vi "TDC_DAQV26_Paralled_muon.vi"(8 "error in (no error)":errorcluster, 9 "stop":bool, 10 "save data":bool=TRUE, 11 "SMA mode":bool=TRUE) -> (3 "rate":dbl=1.039685324035924)   [LabVIEW 2017]
uses:
  <vilib>/Utility/file.llb/Write Delimited Spreadsheet (DBL).vi
  <vilib>/Utility/file.llb/Write Delimited Spreadsheet (I64).vi
panel:
  out "substring 3":string
  out "fine 2":u64=218864601 format="%x"
  out "substring 2":string
  out "concatenated string 2":string="#"
  out "hex integer string 2":string="23"
  out "x-y":i32=35
  out "substring":string
  in  "gps":bool
  out "hex integer string":string="07E8"
  out "Year":string="2024"
  out "error out 3":errorcluster
  in  "factor":i32=128
  in  "displayCR":bool=TRUE
  in  "Counter Setting":dbl=100000.0 format="%#_13g"
  in  "replace dat":bool
  in  "append csv":bool=TRUE
  in  "concatenated string":string="Z\u000f"
  out "number":u32=35
  out "element":string
  out "fine":u64=197 format="%x"
  in  "UDP Config":bool=TRUE
  in  "data  path":path=path "G:/tdc/2017"
  out "cal 2":u64[](graph)
  in  "Thresholds (mV)":u16[](array[numeric])=[580, 580, 580, 580, 600, 600, 600, 600, 580, 580, 600, 600, 600, 600, 600, 600, 580, 580, 600, 600, 600, 600, 600, 600, 580, 580, 600, 600, 600, 600, 600, 600]
  out "error out 2":errorcluster={"status"=TRUE, "code"=1, "source"="Dequeue Element in TDC_DAQV26_Paralled_muon.vi"}
  in  "display":bool=TRUE
  in  "Thresholds":u16=580
  in  "one key for threshold":bool=TRUE
  in  "RST":bool
  in  "通道数量":i32=128
  out "Cal Table":u32[](array[numeric])=[100002, 100002, 100002, 100002, 100002, 100002, 100002, 100002, 100002, 100002, 100002, 100002, 100002, 100002, 100002, 100002, 100002, 100002, 100002, 100002, 100002, 100002, 100002, 100002, 100002, 100002, 100002, 100002, 100002, 100002, 100002, 100002, 100002, 0, 0, 0, 100002, 0, 0, 0, 0, 0, 0, 0, 0, 0, 0, 0, 0, 0, 0, 0, 0, 0, 0, 0, 0, 0, 0, 0, 0, 0, 0, 0, 0, 0, 0, 0, 0, 0, 0, 0, 0, 0, 0, 0, 0, 0, 0, 0, 0, 0, 0, 0, 0, 0, 0, 0, 0, 0, 0, 0, 0, 0, 0, 0, 0, 0, 0, 0, 0, 0, 0, 0, 0, 0, 0, 0, 0, 0, 0, 0, 0, 0, 0, 0, 0, 0, 0, 0, 0, 0, 0, 0, 0, 0, 0, 0]
  in  "channel for cal":i32
  out "channel number":u64=10
  in  "bytes to read":i32=320
  out "Calibration Counter":i32=100000
  out "Event index":i32=97959
  out "cal":u32[](graph)=[0, 0, 0, 0, 0, 0, 0, 0, 0, 0, 0, 0, 0, 0, 0, 0, 0, 0, 0, 0, 0, 0, 0, 0, 0, 0, 0, 0, 0, 0, 0, 0, 0, 0, 0, 0, 0, 0, 0, 0, 0, 0, 0, 0, 0, 0, 0, 0, 0, 0, 0, 0, 0, 0, 0, 0, 0, 0, 0, 0, 0, 0, 0, 0, 0, 0, 0, 0, 0, 0, 0, 0, 0, 0, 0, 0, 0, 0, 0, 0, 0, 0, 0, 0, 0, 0, 0, 0, 0, 0, 0, 0, 0, 0, 0, 0, 0, 0, 0, 0, 0, 0, 0, 0, 0, 0, 0, 0, 0, 0, 0, 0, 0, 0, 0, 0, 0, 0, 0, 0, 0, 0, 0, 0, 0, 0, 0, 0, 0, 0, 0, 0, 0, 0, 0, 0, 0, 0, 0, 0, 0, 0, 0, 0, 0, 0, 0, 0, 0, 0, 0, 0, 0, 0, 0, 0, 0, 0, 0, 10, 71, 320, 55, 788, 157, 172, 696, 64, 82, 262, 173, 135, 530, 87, 255, 177, 53, 608, 293, 326, 71, 47, 118, 254, 336, 311, 104, 51, 60, 101, 372, 166, 178, 168, 245, 175, 255, 440, 146, 44, 45, 205, 363, 299, 66, 85, 64, 46, 161, 73, 87, 47, 79, 666, 246, 61, 75, 55, 178, 83, 250, 291, 46, 49, 206, 160, 459, 68, 164, 175, 127, 374, 157, 65, 63, 140, 125, 65, 81, 86, 171, 166, 294, 130, 57, 56, 35, 61, 101, 38, 351, 101, 459, 108, 74, 68, 117, 70, 135, 136, 194, 46, 513, 47, 37, 299, 54, 123, 69, 303, 46, 39, 36, 153, 122, 350, 130, 86, 162, 135, 148, 117, 311, 184, 79, 167, 252, 57, 123, 76, 268, 69, 54, 100, 252, 57, 39, 66, 495, 175, 138, 53, 162, 69, 123, 49, 63, 111, 337, 184, 50, 101, 59, 156, 75, 54, 232, 351, 53, 241, 137, 45, 169, 83, 112, 45, 278, 398, 106, 103, 61, 225, 114, 53, 349, 136, 144, 139, 230, 47, 41, 39, 128, 264, 88, 328, 63, 460, 373, 100, 51, 59, 290, 101, 576, 134, 101, 92, 70, 72, 60, 138, 192, 163, 185, 250, 92, 55, 83, 85, 80, 179, 133, 107, 81, 386, 79, 65, 147, 96, 111, 306, 281, 141, 140, 234, 96, 322, 73, 54, 60, 107, 284, 77, 115, 71, 69, 168, 320, 56, 166, 190, 154, 153, 95, 120, 232, 147, 59, 47, 78, 316, 84, 44, 84, 412, 156, 67, 173, 188, 56, 93, 78, 172, 586, 79, 69, 63, 47, 30, 64, 176, 76, 99, 504, 173, 60, 57, 150, 175, 76, 54, 70, 88, 41, 519, 208, 91, 467, 49, 53, 40, 46, 371, 122, 142, 66, 216, 120, 48, 56, 64, 174, 362, 68, 302, 82, 78, 72, 347, 92, 85, 188, 270, 100, 62, 123, 182, 178, 324, 127, 165, 107, 189, 184, 56, 252, 122, 111, 123, 54, 240, 39, 50, 87, 353, 187, 265, 56, 49, 52, 48, 128, 342, 202, 83, 124, 111, 57, 70, 215, 119, 215, 90, 61, 159, 220, 46, 92, 225, 254, 104, 89, 54, 63, 93, 57, 49, 59, 794, 66, 46, 60, 66, 62, 331, 151, 145, 387, 94, 133, 45, 205, 163, 301, 70, 138, 341, 53, 361, 46, 47, 68, 64, 302, 126, 52, 31, 77, 86, 107, 236, 304, 50, 48, 82, 126, 116, 287, 66, 89, 80, 166, 51, 64, 238, 179, 185, 64, 408, 113, 149, 102, 141, 66, 247, 73, 343, 243, 108, 99, 64, 283, 309, 137, 95, 347, 128, 229, 519, 63, 378, 71, 121, 342, 558, 83, 91, 138, 114, 155, 93, 202, 215, 179, 311, 80, 108, 142, 151, 209, 117, 114, 100, 128, 194, 185, 423, 207, 173, 217, 105, 119, 114, 321, 92, 139, 114, 73, 159, 67, 91, 311, 77, 144, 150, 323, 241, 221, 146, 174, 293, 75, 57, 79, 130, 288, 72, 123, 113, 361, 224, 84, 135, 88, 118, 155, 184, 119, 62, 88, 114, 62, 186, 97, 52, 234, 165, 49, 71, 72, 195, 364, 217, 84, 63, 64, 73, 162, 227, 133, 507, 60, 197, 272, 61, 49, 160, 197, 89, 89, 128, 107, 117, 177, 163, 91, 114, 57, 64, 219, 83, 119, 170, 56, 77, 56, 67, 218, 120, 281, 171, 136, 159, 61, 43, 105, 74, 126, 202, 159, 98, 320, 66, 105, 324, 210, 151, 79, 81, 115, 144, 148, 470, 209, 115, 114, 121, 116, 138, 158, 349, 112, 170, 362, 161, 214, 209, 170, 130, 131, 389, 42, 175, 208, 68, 128, 313, 195, 123, 303, 45, 253, 76, 73, 95, 254, 197, 55, 99, 114, 169, 141, 377, 223, 106, 53, 121, 137, 49, 56, 57, 46, 138, 258, 58, 83, 123, 67, 62, 147, 76, 33, 67, 174, 25, 16, 19, 20, 39, 20, 82, 17, 24, 72, 21, 8, 21, 21, 10, 2, 6, 6, 3, 0, 2, 0, 0, 0, 0, 0, 0, 0, 0, 0, 0, 0, 0, 0, 0, 0, 0, 0, 0, 0, 0, 0, 0, 0, 0, 0, 0, 0, 0, 0, 0, 0, 0, 0, 0, 0, 0, 0, 0, 0, 0, 0, 0, 0, 0, 0, 0, 0, 0, 0, 0, 0, 0, 0, 0, 0, 0, 0, 0, 0, 0, 0, 0, 0, 0, 0, 0, 0, 0, 0, 0, 0, 0, 0, 0, 0, 0, 0, 0, 0, 0, 0, 0, 0, 0, 0, 0, 0, 0, 0, 0, 0, 0, 0, 0, 0, 0, 0, 0, 0, 0, 0, 0, 0, 0, 0, 0, 0, 0, 0, 0, 0, 0, 0, 0, 0, 0, 0, 0, 0, 0, 0, 0, 0, 0, 0, 0, 0, 0, 0, 0, 0, 0, 0, 0, 0, 0, 0, 0, 0, 0, 0, 0, 0, 0, 0, 0, 0, 0, 0, 0, 0, 0, 0, 0, 0, 0, 0, 0, 0, 0, 0, 0, 0, 0, 0, 0, 0, 0, 0, 0, 0, 0, 0, 0, 0, 0, 0, 0, 0, 0, 0, 0, 0, 0, 0, 0, 0, 0, 0, 0, 0, 0, 0, 0, 0, 0, 0, 0, 0, 0, 0, 0, 0, 0, 0, 0, 0, 0, 0, 0, 0, 0, 0, 0, 0, 0, 0, 0, 0, 0, 0, 0, 0, 0, 0, 0, 0, 0, 0, 0, 0, 0, 0, 0, 0, 0, 0, 0, 0, 0, 0, 0, 0, 0, 0, 0, 0, 0, 0, 0, 0, 0, 0, 0, 0, 0, 0, 0, 0, 0, 0, 0, 0, 0, 0, 0, 0, 0, 0, 0, 0, 0, 0, 0, 0, 0, 0, 0, 0, 0, 0, 0, 0, 0, 0, 0, 0, 0, 0, 0, 0, 0, 0, 0, 0, 0, 0, 0, 0, 0, 0, 0, 0, 0, 0, 0, 0, 0, 0, 0, 0, 0, 0, 0, 0, 0, 0, 0, 0, 0, 0, 0, 0, 0, 0, 0, 0, 0, 0, 0, 0, 0, 0, 0, 0, 0, 0, 0, 0, 0, 0, 0, 0, 0, 0, 0, 0, 0, 0, 0, 0, 0, 0, 0, 0, 0, 0, 0, 0, 0, 0, 0, 0, 0, 0, 0, 0, 0, 0, 0, 0, 0, 0, 0, 0, 0, 0, 0, 0, 0, 0, 0, 0, 0, 0, 0, 0, 0, 0, 0, 0, 0, 0, 0, 0, 0, 0, 0, 0, 0, 0, 0, 0, 0, 0, 0, 0, 0, 0, 0, 0, 0, 0, 0, 0, 0, 0, 0, 0, 0, 0, 0, 0, 0, 0, 0, 0, 0, 0, 0, 0, 0, 0, 0, 0, 0, 0, 0, 0, 0, 0, 0, 0, 0, 0, 0, 0, 0, 0, 0, 0, 0, 0, 0, 0, 0, 0, 0, 0, 0, 0, 0, 0, 0, 0, 0, 0, 0, 0, 0, 0, 0, 0, 0, 0, 0, 0, 0, 0, 0, 0, 0, 0, 0, 0, 0, 0, 0, 0, 0, 0, 0, 0, 0, 0, 0, 0, 0, 0, 0, 0, 0, 0, 0, 0, 0, 0, 0, 0, 0, 0, 0, 0, 0, 0, 0, 0, 0, 0, 0, 0, 0, 0, 0, 0, 0, 0, 0, 0, 0, 0, 0, 0, 0, 0, 0, 0, 0, 0, 0, 0, 0, 0, 0, 0, 0, 0, 0, 0, 0, 0, 0, 0, 0, 0, 0, 0, 0, 0, 0, 0, 0, 0, 0, 0, 0, 0, 0, 0, 0, 0, 0, 0, 0, 0, 0, 0, 0, 0, 0, 0, 0, 0, 0, 0, 0, 0, 0, 0, 0, 0, 0, 0, 0, 0, 0, 0, 0, 0, 0, 0, 0, 0, 0, 0, 0, 0, 0, 0, 0, 0, 0, 0, 0, 0, 0, 0, 0, 0, 0, 0, 0, 0, 0, 0, 0, 0, 0, 0, 0, 0, 0, 0, 0, 0, 0, 0, 0, 0, 0, 0, 0, 0, 0, 0, 0, 0, 0, 0, 0, 0, 0, 0, 0, 0, 0, 0, 0, 0, 0, 0, 0, 0, 0, 0, 0, 0, 0, 0, 0, 0, 0, 0, 0, 0, 0, 0, 0, 0, 0, 0, 0, 0, 0, 0, 0, 0, 0, 0, 0, 0, 0, 0, 0, 0, 0, 0, 0, 0, 0, 0, 0, 0, 0, 0, 0, 0, 0, 0, 0, 0, 0, 0, 0, 0, 0, 0, 0, 0, 0, 0, 0, 0, 0, 0, 0, 0, 0, 0, 0, 0, 0, 0, 0, 0, 0, 0, 0, 0, 0, 0, 0, 0, 0, 0, 0, 0, 0, 0, 0, 0, 0, 0, 0, 0, 0, 0, 0, 0, 0, 0, 0, 0, 0, 0, 0, 0, 0, 0, 0, 0, 0, 0, 0, 0, 0, 0, 0, 0, 0, 0, 0, 0, 0, 0, 0, 0, 0, 0, 0, 0, 0, 0, 0, 0, 0, 0, 0, 0, 0, 0, 0, 0, 0, 0, 0, 0, 0, 0, 0, 0, 0, 0, 0, 0, 0, 0, 0, 0, 0, 0, 0, 0, 0, 0, 0, 0, 0, 0, 0, 0, 0, 0, 0, 0, 0, 0, 0, 0, 0, 0, 0, 0, 0, 0, 0, 0, 0, 0, 0, 0, 0, 0, 0, 0, 0, 0, 0, 0, 0, 0, 0, 0, 0, 0, 0, 0, 0, 0, 0, 0, 0, 0, 0, 0, 0, 0, 0, 0, 0, 0, 0, 0, 0, 0, 0, 0, 0, 0, 0, 0, 0, 0, 0, 0, 0, 0, 0, 0, 0, 0, 0, 0, 0, 0, 0, 0, 0, 0, 0, 0, 0, 0, 0, 0, 0, 0, 0, 0, 0, 0, 0, 0, 0, 0, 0, 0, 0, 0, 0, 0, 0, 0, 0, 0, 0, 0, 0, 0, 0, 0, 0, 0, 0, 0, 0, 0, 0, 0, 0, 0, 0, 0, 0, 0, 0, 0, 0, 0, 0, 0, 0, 0, 0, 0, 0, 0, 0, 0, 0, 0, 0, 0, 0, 0, 0, 0, 0, 0, 0, 0, 0, 0, 0, 0, 0, 0, 0, 0, 0, 0, 0, 0, 0, 0, 0, 0, 0, 0, 0, 0, 0, 0, 0, 0, 0, 0, 0, 0, 0, 0, 0, 0, 0, 0, 0, 0, 0, 0, 0, 0, 0, 0, 0, 0, 0, 0, 0, 0, 0, 0, 0, 0, 0, 0, 0, 0, 0, 0, 0, 0, 0, 0, 0, 0, 0, 0, 0, 0, 0, 0, 0, 0, 0, 0, 0, 0, 0, 0, 0, 0, 0, 0, 0, 0, 0, 0, 0, 0, 0, 0, 0, 0, 0, 0, 0, 0, 0, 0, 0, 0, 0, 0, 0, 0, 0, 0, 0, 0, 0, 0, 0, 0, 0, 0, 0, 0, 0, 0, 0, 0, 0, 0, 0, 0, 0, 0, 0, 0, 0, 0, 0, 0, 0, 0, 0, 0, 0, 0, 0, 0, 0, 0, 0, 0, 0, 0, 0, 0, 0, 0, 0, 0, 0, 0, 0, 0, 0, 0, 0, 0, 0, 0, 0, 0, 0, 0, 0, 0, 0, 0, 0, 0, 0, 0, 0, 0, 0, 0, 0, 0, 0, 0, 0, 0, 0, 0, 0, 0, 0, 0, 0, 0, 0, 0, 0, 0, 0, 0, 0, 0, 0, 0, 0, 0, 0, 0, 0, 0, 0, 0, 0, 0, 0, 0, 0, 0, 0, 0, 0, 0, 0, 0, 0, 0, 0, 0, 0, 0, 0, 0, 0, 0, 0, 0, 0, 0, 0, 0, 0, 0, 0]
  out "error out":errorcluster
  out "appended path":path=path "G:/tdc/2017/test_20241217_115315.dat"
  in  "filename":string="test"
  in  "Events":i32=110000 min=1
  in  "timeout (ms)":i32=10000
  in  "address":string="192.168.10.35"
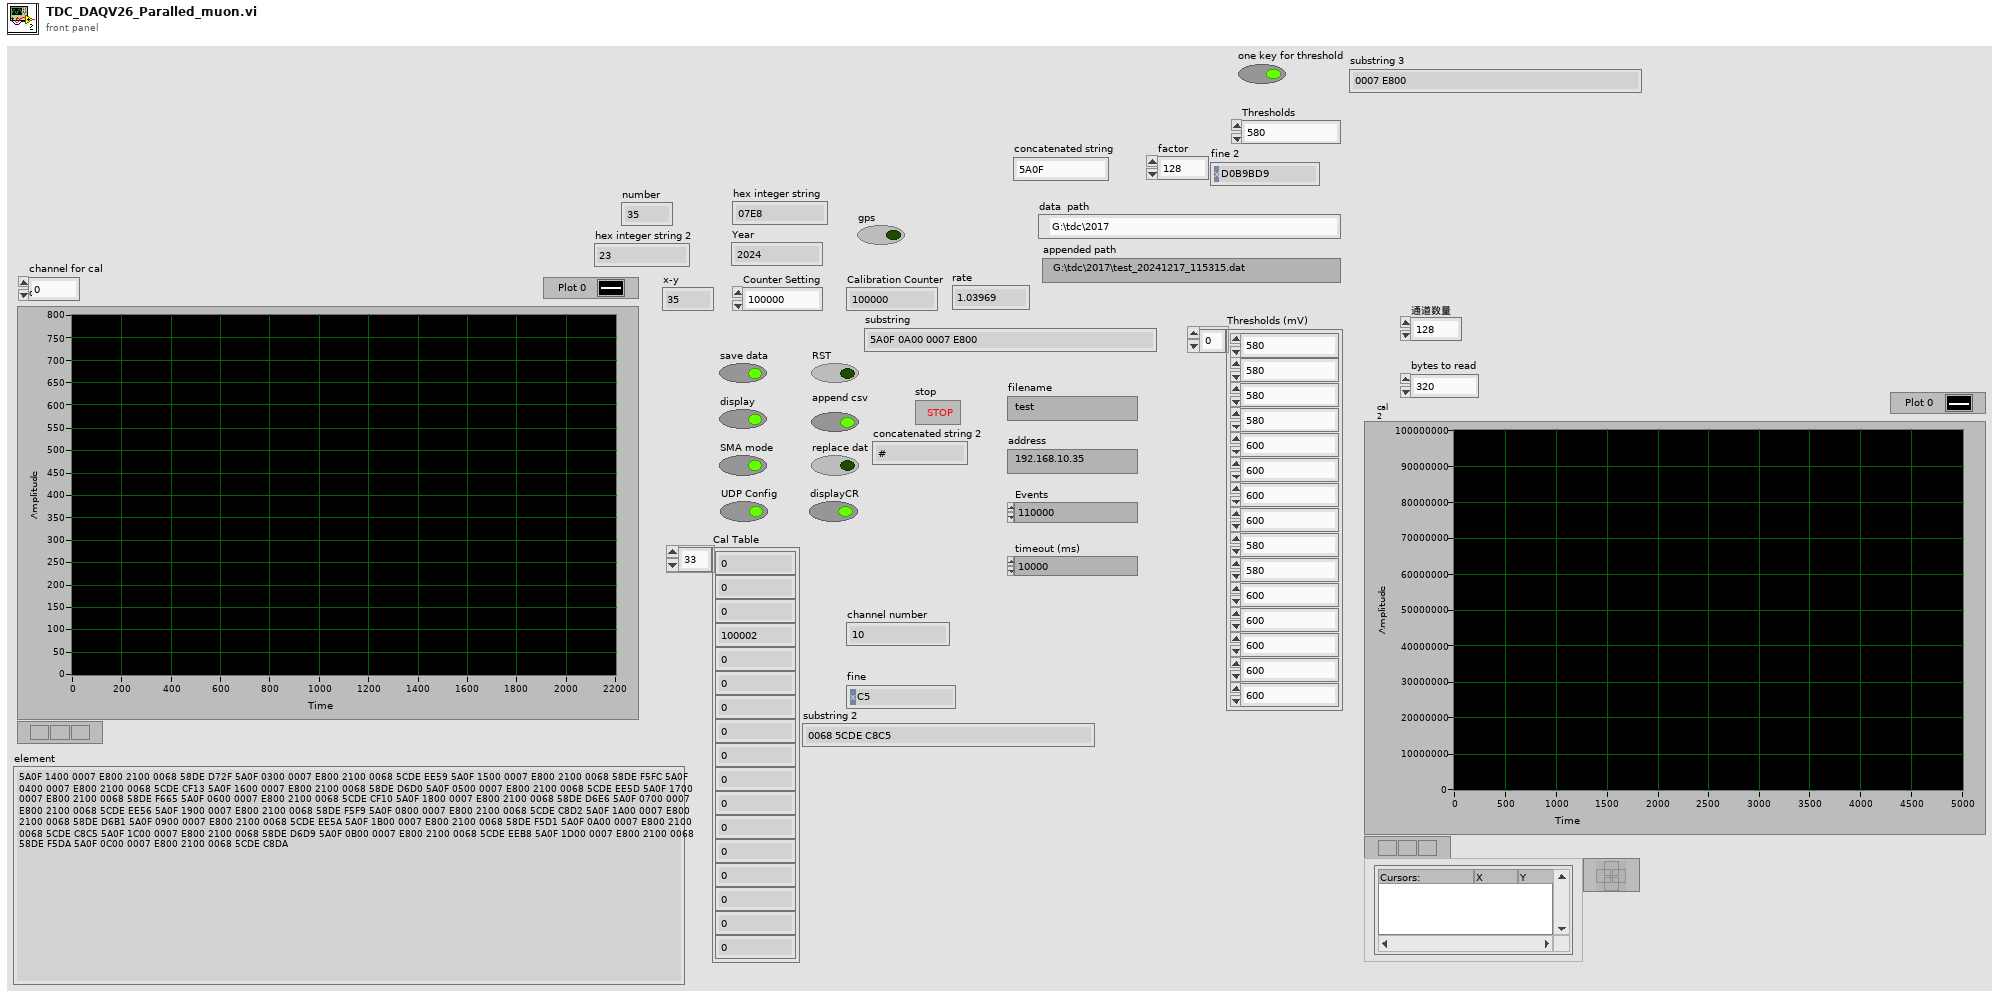
[diagram p1: front panel]
types:
  T1 = enum16{"open", "replace", "create", "open or create", "replace or create", "replace or create with confirmation"}
  T2 = enum16{"Standard", "Buffered", "CRLF", "Immediate"}
  T3 = enum16{"big-endian, network order", "native, host order", "little-endian"}
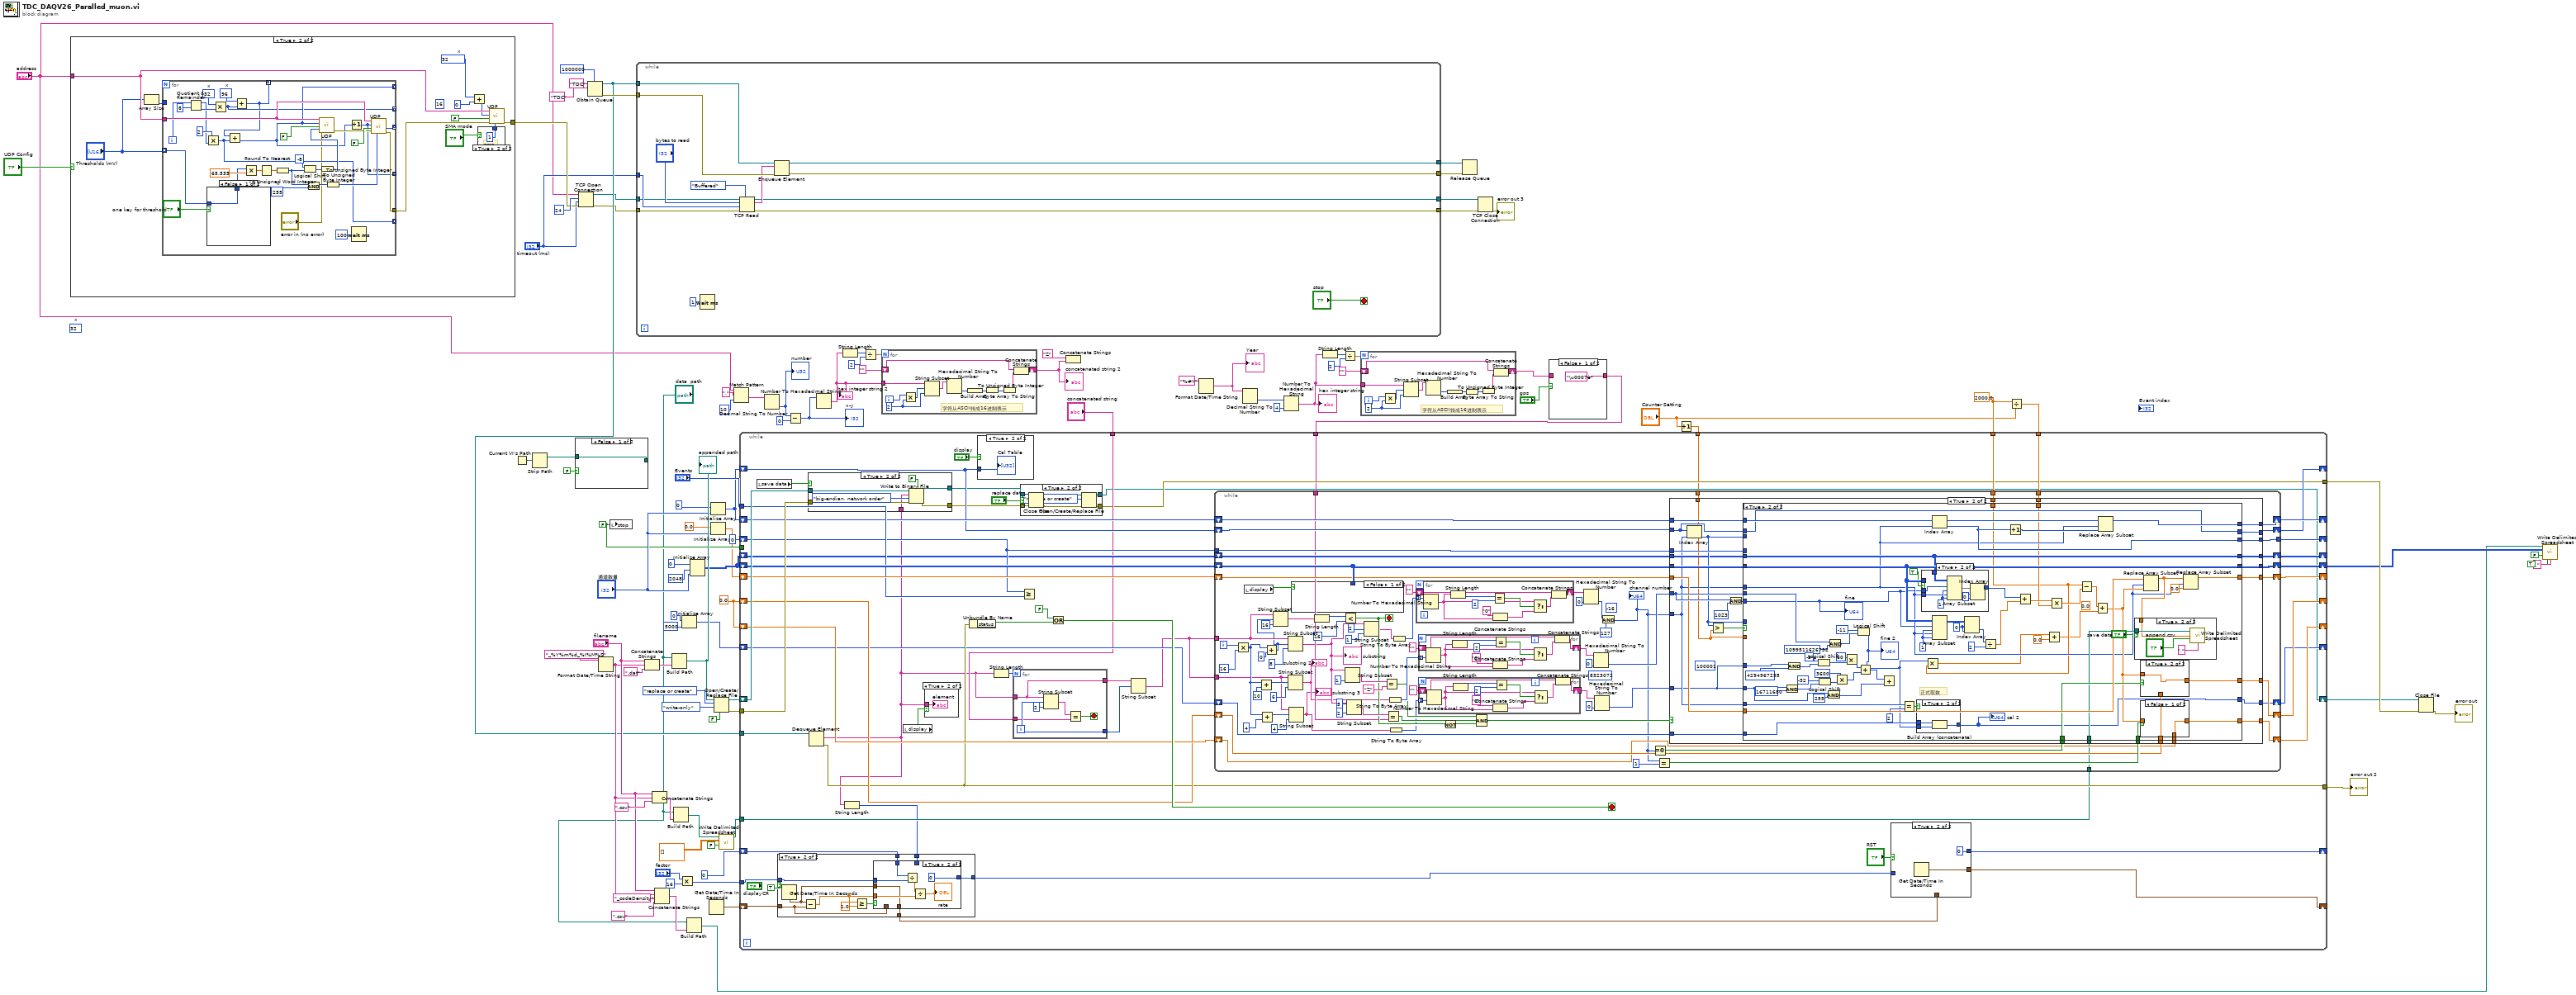
[diagram p0: block diagram]
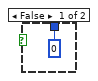
[diagram p4: hidden frame]
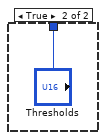
[diagram p5: hidden frame]
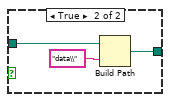
[diagram p6: hidden frame]
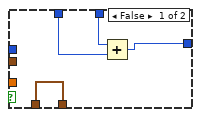
[diagram p11: hidden frame]
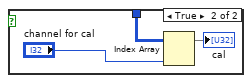
[diagram p14: hidden frame]
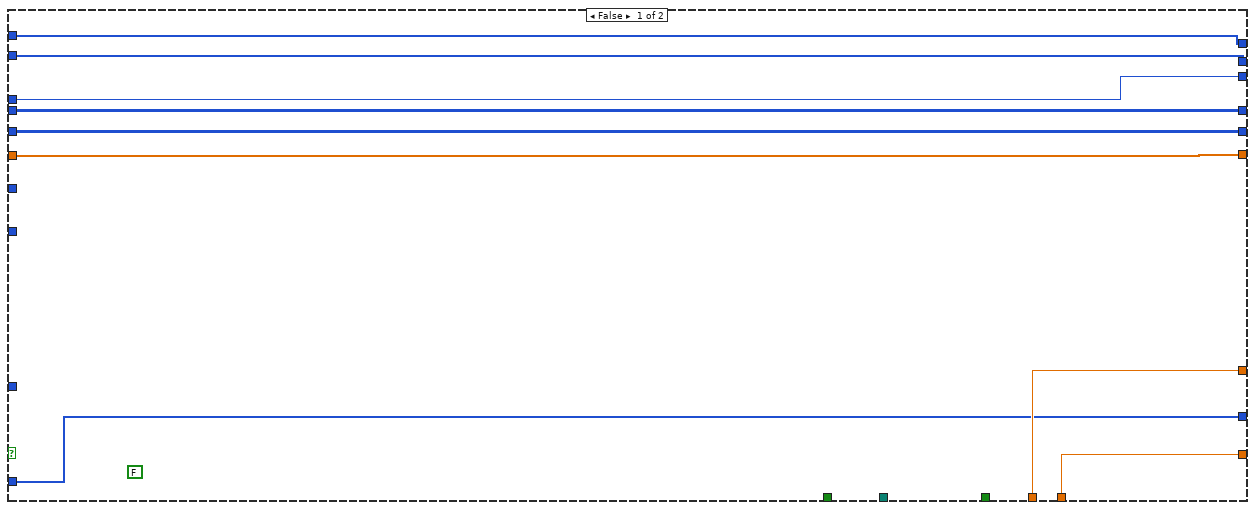
[diagram p15: hidden frame]
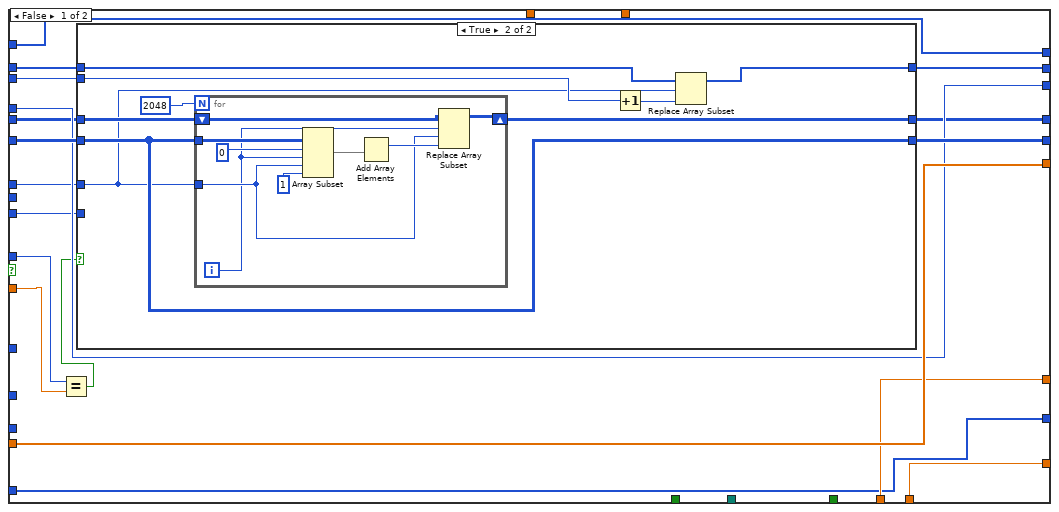
[diagram p16: hidden frame]
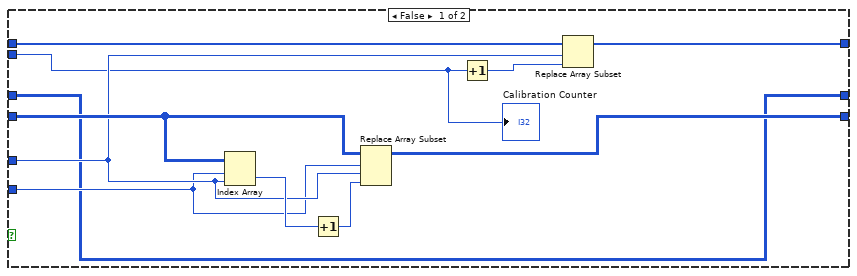
[diagram p17: hidden frame]
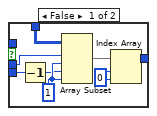
[diagram p20: hidden frame]
diagram:
  w26 = 2000.0 ("x")
  (unwired) u16 32  # x
  w68 = FALSE ("stop")
  w78 = 0.0
  n1 = case shown="True" "UDP Config" {
    tunnel: "address" -> [_ w111]
    tunnel: [_ w108] -> w69
    frame False {
    }
    frame True {
      (unwired) u32 16 ("Address")
      w102 = u16 32  # x
      n2 = Array Size(array="Thresholds (mV)") -> (size(s)=w105:i32)
      n3 = for {
        tunnel: w111 -> [w141]
        tunnel: "Thresholds (mV)" -> [w127] mode=indexing
        tunnel: [w135] -> _ mode=indexing
        tunnel: [w130] -> w109
        tunnel: w105 -> [_]
        tunnel: [w121] -> _ mode=indexing
        tunnel: [w120] -> _ mode=indexing
        tunnel: [w119] -> _ mode=indexing
        tunnel: [w118] -> _ mode=indexing
        tunnel: [w117] -> _ mode=indexing
        i -> [w122]
        w123 = u16 96  # x
        w124 = u16 32  # x
        w137 = u16 255  # x
        n4 = Quotient & Remainder(x=w122, y=8) -> (x-y*floor(x/y)=w116:i32, floor(x/y)=w125:i32)
        n5 = Multiply(x=2, y=w116) -> (x*y=w117:i32)
        n6 = case shown="False" "one key for threshold" {
          tunnel: [w147 "Thresholds"] -> w128
          tunnel: w127 -> [w147 _]
          frame False {
          }
          frame True {
          }
        }
        n7 = Multiply(x=w124, y=w125) -> (x*y=w119:i32)
        n8 = Add(x=w123, y=w119) -> (x+y=w118:i32)
        n9 = Add(x=w118, y=w117) -> (x+y=w121:i32)
        n10 = Multiply(x=w128, y=65.535) -> (x*y=w144:dbl)
        n11 = Round To Nearest(number=w144) -> (nearest integer value=w142:dbl)
        n12 = To Unsigned Word Integer(number=w142) -> (unsigned 16bit integer=w132:u16)
        n13 = Logical Shift(y=i16 -8, x=w132) -> (x << y=w139:u16)
        n14 = And(x=w132, y=w137) -> (x .and. y?=w136:u16)
        n15 = To Unsigned Byte Integer(number=w139) -> (unsigned 8bit integer=w138:u8)
        n16 = call "UDP.vi"("In"=w138, "error in (no error)"="error in (no error)", "Read (TRUE)"=FALSE, "Address"=w121, "IP address"=w141) -> ("error out"=w131:errorcluster)  [unwired: 4 in, 1 out]
        n17 = To Unsigned Byte Integer(number=w136) -> (unsigned 8bit integer=w134:u8)
        n18 = Increment(x=w121) -> (x+1=w120:i32)
        n19 = Wait (ms)(milliseconds to wait=u32 100) -> ()  [unwired: 1 out]
        n20 = call "UDP.vi"("In"=w134, "error in (no error)"=w131, "Read (TRUE)"=FALSE, "Address"=w120, "IP address"=w141) -> ("error out"=w130:errorcluster, "Out"=w135:u8)  [unwired: 4 in]
      }
      n21 = Add(x=w102, y=u32 0 ("Address")) -> (x+y=w101:u32)
      n22 = case shown="True" "SMA mode" {
        tunnel: [u8 0 ("In") u8 1 ("In")] -> w107
        frame False {
        }
        frame True {
          # "sma"
        }
      }
      n23 = call "UDP.vi"("In"=w107, "error in (no error)"=w109, "Read (TRUE)"=FALSE, "Address"=w101, "IP address"=w111) -> ("error out"=w108:errorcluster)  [unwired: 4 in, 1 out]
    }
  }
  n24 = Current VI's Path() -> (path=w94:path)
  n25 = Strip Path(path=w94) -> (stripped path=w93:path)  [unwired: 1 out]
  n26 = case shown="False" FALSE {
    tunnel: w93 -> [w149 w151]
    tunnel: [w149 w150] -> _
    frame False {
    }
    frame True {
      n27 = Build Path(base path=w151, name or relative path="data\\") -> (appended path=w150:path)
    }
  }
  n28 = TCP Open Connection(address="address", remote port or service name=u16 24 ("port"), timeout ms (60000)="timeout (ms)", error in (no error)=w69) -> (connection ID=w52:refnum<k5>, error out=w53:errorcluster)  [unwired: 1 in]
  n29 = Obtain Queue(max queue size (-1, unlimited)=1000000, name (unnamed)="TDC", element data type="TDC" ("name (unnamed)")) -> (queue out=w54:refnum<queue>, error out=w55:errorcluster)  [unwired: 2 in, 1 out]
  n30 = Format Date/Time String(time format string (%c)="_%Y%m%d_%I%M%S") -> (date/time string=w66:string)  [unwired: 2 in]
  n31 = local write "stop"(w68) -> ()
  n32 = while {
    tunnel: w54 -> [w166]
    tunnel: w55 -> [w165]
    tunnel: w53 -> [w163]
    tunnel: "timeout (ms)" -> [w162]
    tunnel: w52 -> [w161]
    tunnel: [w159] -> w51
    tunnel: [w158] -> w50
    tunnel: [w156] -> w49
    tunnel: [w155] -> w48
    stop <- "stop" stop-if-true
    n33 = Wait (ms)(milliseconds to wait=u32 1) -> ()  [unwired: 1 out]
    n34 = TCP Read(connection ID=w161, bytes to read="bytes to read", error in (no error)=w163, 7:T2."Buffered" ("mode (standard)"), 9:w162) -> (connection ID out=w159:refnum<k5>, data out=w160:string, error out=w158:errorcluster)
    n35 = Enqueue Element(queue=w166, element=w160, error in (no error)=w165) -> (queue out=w156:refnum<queue>, error out=w155:errorcluster)  [unwired: 1 in, 1 out]
  }
  n36 = Concatenate Strings("filename", w66, ".dat") -> (w92:string)
  n37 = Concatenate Strings("filename", w66, ".csv") -> (w80:string)
  n38 = Concatenate Strings("filename", w66, "_codeDensity" ("string"), ".csv") -> (w63:string)
  n39 = Build Path(base path="data  path", name or relative path=w92) -> (appended path=w91:path)
  "appended path" <- w91
  n40 = Build Path(base path="data  path", name or relative path=w80) -> (appended path=w75:path)
  n41 = Multiply(x="factor", y=16) -> (x*y=w19:i32)
  n42 = Initialize Array(u32 0 ("element"), 5000 ("dimension size")) -> (w42:u32[])
  n43 = Build Path(base path="data  path", name or relative path=w63) -> (appended path=w60:path)
  n44 = Initialize Array(u32 0 ("element"), 2048 ("dimension size"), "通道数量") -> (w77:u32[][])
  n45 = Get Date/Time In Seconds() -> (seconds since 1Jan1904=w70:timestamp)
  n46 = Initialize Array(u32 0 ("element"), "通道数量") -> (w79:u32[])
  n47 = Initialize Array(0.0, "通道数量") -> (w44:dbl[])
  n48 = Open/Create/Replace File(file path (use dialog)=w91, operation (0:open)=T1."replace or create", access (0:read/write)=enum16{"read/write", "read-only", "write-only"}."write-only", disable buffering (F)=FALSE) -> (refnum out=w96:refnum<file>, error out=w95:errorcluster)  [unwired: 2 in, 1 out]
  n49 = call-poly <vilib>:"Write Delimited Spreadsheet.vi"("file path (dialog if empty)"=w75, "2D data"=dbl[][] [], "append to file? (new file:F)"=FALSE) -> ("new file path (Not A Path if cancelled)"=w74:path)  [unwired: 11 in, 1 out]
  n50 = Match Pattern(string="address", regular expression="." ("search string"), offset (0)=10) -> (after substring=w31:string)  [unwired: 3 out]
  n51 = Decimal String To Number(string=w31) -> (number=w3:i32)  [unwired: 2 in, 1 out]
  "number" <- w3
  n52 = Subtract(x=w3, y=0) -> (x-y=w2:i32)
  "x-y" <- w2
  n53 = Number To Hexadecimal String(2:w2) -> (0:w29:string)  [unwired: 1 in]
  "hex integer string 2" <- w29
  n54 = String Length(string=w29) -> (length=w36:i32)
  n55 = Divide(x=w36, y=2) -> (x/y=w37:dbl)
  n56 = for {
    N: w37 -> [_]
    shift-right: [w177] -> w1
    shift-left: "" ("format string") -> [w176]
    tunnel: w29 -> [w167]
    i -> [w175]
    w169 = 2 ("y")
    # "字符从ASCII转成16进制表示"
    n57 = Multiply(x=w175, y=w169) -> (x*y=w168:i32)
    n58 = String Subset(string=w167, offset (0)=w168, length (rest)=w169) -> (substring=w170:string)
    n59 = Hexadecimal String To Number(string=w170) -> (number=w174:u32)  [unwired: 2 in, 1 out]
    n60 = Build Array(w174) -> (w173:u32[])
    n61 = To Unsigned Byte Integer(number=w173) -> (unsigned 8bit integer=w172:u8[])
    n62 = Byte Array To String(unsigned byte array=w172) -> (string=w171:string)
    n63 = Concatenate Strings(w176, w171) -> (w177:string)
  }
  "concatenated string 2" <- w1
  n64 = Concatenate Strings("Z", w1) -> ()  [unwired: 1 out]
  n65 = Format Date/Time String(time format string (%c)="%#Y") -> (date/time string=w15:string)  [unwired: 2 in]
  "Year" <- w15
  n66 = Decimal String To Number(string=w15) -> (number=w14:i32)  [unwired: 2 in, 1 out]
  n67 = Number To Hexadecimal String(1:i16 4 ("width (-)"), 2:w14) -> (0:w8:string)
  "hex integer string" <- w8
  n68 = String Length(string=w8) -> (length=w10:i32)
  n69 = Divide(x=w10, y=2) -> (x/y=w11:dbl)
  n70 = for {
    N: w11 -> [_]
    shift-right: [w188] -> w7
    shift-left: "" ("format string") -> [w187]
    tunnel: w8 -> [w178]
    i -> [w186]
    w180 = 2 ("y")
    # "字符从ASCII转成16进制表示"
    n71 = Multiply(x=w186, y=w180) -> (x*y=w179:i32)
    n72 = String Subset(string=w178, offset (0)=w179, length (rest)=w180) -> (substring=w181:string)
    n73 = Hexadecimal String To Number(string=w181) -> (number=w185:u32)  [unwired: 2 in, 1 out]
    n74 = Build Array(w185) -> (w184:u32[])
    n75 = To Unsigned Byte Integer(number=w184) -> (unsigned 8bit integer=w183:u8[])
    n76 = Byte Array To String(unsigned byte array=w183) -> (string=w182:string)
    n77 = Concatenate Strings(w187, w182) -> (w188:string)
  }
  n78 = Release Queue(queue=w49, error in (no error)=w48) -> ()  [unwired: 1 in, 3 out]
  n79 = TCP Close Connection(connection ID=w51, error in (no error)=w50) -> (error out=→"error out 3":errorcluster)  [unwired: 1 in, 1 out]
  n80 = case shown="False" "gps" {
    tunnel: w7 -> [_ w190]
    tunnel: ["\u0007è" ("format string") w190] -> w6
    frame False {
    }
    frame True {
    }
  }
  n81 = Increment(x="Counter Setting") -> (x+1=w22:dbl)
  n82 = Divide(x=w26, y="Counter Setting") -> (x/y=w25:dbl)
  n83 = while {
    tunnel: w95 -> [w245]
    tunnel: [w219] -> w47
    tunnel: [w203] -> w88
    shift-right: [w242] -> w61
    shift-left: w77 -> [w243]
    shift-right: [w228] -> _
    shift-left: w44 -> [w241]
    tunnel: "Events" -> [w239]
    shift-right: [w238] -> _
    shift-left: w79 -> [w237]
    shift-right: [w236] -> _
    shift-left: u32 0 ("element") -> [w235]
    shift-right: [w234] -> _
    shift-left: w79 -> [w221]
    shift-right: [w233] -> _
    shift-left: w78 -> [w230]
    shift-right: [w232] -> _
    shift-left: w78 -> [w231]
    shift-right: [w223] -> _
    shift-left: w77 -> [w229]
    tunnel: w74 -> [w215]
    shift-right: [w227] -> _
    shift-left: 0 -> [w197]
    shift-right: [w225] -> _
    shift-left: w70 -> [w224]
    tunnel: w68 -> [_]
    tunnel: w54 -> [w220]
    shift-right: [w216] -> _
    shift-left: w42 -> [w217]
    tunnel: "concatenated string" -> [w211]
    tunnel: w26 -> [w209]
    tunnel: w25 -> [w208]
    shift-right: [w202] -> w24
    shift-left: w96 -> [w244]
    tunnel: w22 -> [w201]
    tunnel: w19 -> [w194]
    tunnel: w6 -> [w191]
    stop <- w240 stop-if-true
    n84 = local read "save data"() -> (w196:bool)
    n85 = Dequeue Element(queue=w220) -> (element=w207:string, error out=w219:errorcluster)  [unwired: 2 in, 2 out]
    n86 = case shown="True" w196 {
      tunnel: w245 -> [w247 w255]
      tunnel: w244 -> [w248 w254]
      tunnel: w207 -> [_ w251]
      tunnel: [w248 w250] -> w206
      tunnel: [w247 w249] -> w204
      frame False {
      }
      frame True {
        n87 = Write to Binary File(file (use dialog)=w254, data=w251, error in=w255, 5:FALSE ("prepend array or string size? (T)"), 9:T3."big-endian, network order" ("byte order (0:big-endian, network order)")) -> (refnum out=w250:refnum<file>, error out=w249:errorcluster)  [unwired: 1 in, 1 out]
      }
    }
    n88 = String Length(string=w207) -> (length=w198:i32)
    n89 = case shown="True" TRUE {
      tunnel: w224 -> [w272 w277]
      tunnel: [w272 w278] -> w200
      tunnel: w197 -> [w271 w276]
      tunnel: w198 -> [_ w275]
      tunnel: [w271 w274] -> w199
      tunnel: w194 -> [_ w273]
      frame False {
      }
      frame True {
        n90 = Get Date/Time In Seconds() -> (seconds since 1Jan1904=w279:timestamp)
        n91 = Subtract(x=w279, y=w277) -> (x-y=w281:dbl)
        n92 = Greater Or Equal?(x=w281, y=1.0) -> (x >= y?=w282:bool)
        n93 = case shown="True" w282 {
          tunnel: w281 -> [_ w293]
          tunnel: w279 -> [_ w291]
          tunnel: [w286 w291] -> w278
          tunnel: w277 -> [w286 _]
          tunnel: w276 -> [w285 w288]
          tunnel: w275 -> [w284 _]
          tunnel: [w283 0] -> w274
          tunnel: w273 -> [_ w287]
          frame False {
            n94 = Add(x=w284, y=w285) -> (x+y=w283:i32)
          }
          frame True {
            n95 = Divide(x=w288, y=w287) -> (x/y=w290:dbl)
            n96 = Divide(x=w290, y=w293) -> (x/y=→"rate":dbl)
          }
        }
      }
    }
    n97 = local read "display"() -> (w195:bool)
    n98 = case shown="True" w195 {
      tunnel: w207 -> [_ w246]
      frame False {
      }
      frame True {
        "element" <- w246
      }
    }
    n99 = Unbundle By Name(w219) -> ("status"=w218:bool)
    n100 = case shown="True" "display" {
      tunnel: w221 -> [_ w294]
      frame False {
      }
      frame True {
        "Cal Table" <- w294
      }
    }
    n101 = String Length(string=w207) -> (length=w214:i32)
    n102 = for {
      N: w214 -> [_]
      tunnel: w207 -> [w267]
      tunnel: [w267] -> w213
      tunnel: [w266] -> w212
      tunnel: w211 -> [w265]
      i -> [w266]
      stop <- w268 stop-if-true
      n103 = String Subset(string=w267, offset (0)=w266, length (rest)=2 ("length (rest)")) -> (substring=w269:string)
      n104 = Equal?(x=w269, y=w265) -> (x = y?=w268:bool)
    }
    n105 = case shown="True" "replace dat" {
      tunnel: w206 -> [w257 w263]
      tunnel: [w257 w262] -> w202
      tunnel: w204 -> [w256 w259]
      tunnel: [w256 w258] -> w203
      frame False {
      }
      frame True {
        n106 = Close File(refnum=w263, error in=w259) -> (path=w264:path, error out=w260:errorcluster)
        n107 = Open/Create/Replace File(file path (use dialog)=w264, error in=w260, operation (0:open)=T1."replace or create") -> (refnum out=w262:refnum<file>, error out=w258:errorcluster)  [unwired: 3 in, 1 out]
      }
    }
    n108 = Greater Or Equal?(x=w235, y=w239) -> ()  [unwired: 1 out]
    n109 = Or(x=FALSE, y=w218) -> (x .or. y?=w240:bool)
    n110 = String Subset(string=w213, offset (0)=w212) -> (substring=w192:string)  [unwired: 1 in]
    n111 = while {
      tunnel: w192 -> [w325]
      shift-right: [w373] -> w242
      shift-left: w243 -> [w371]
      shift-right: [w369] -> w228
      shift-left: w241 -> [w370]
      shift-right: [w366] -> w238
      shift-left: w237 -> [w365]
      tunnel: [w364] -> w236
      tunnel: w235 -> [w363]
      shift-right: [w361] -> w234
      shift-left: w221 -> [w362]
      shift-right: [w357] -> w233
      shift-left: w230 -> [w355]
      shift-right: [w353] -> w232
      shift-left: w231 -> [w354]
      tunnel: w215 -> [w352]
      shift-right: [w351] -> w223
      shift-left: w229 -> [w319]
      shift-right: [w348] -> w216
      shift-left: w217 -> [w349]
      tunnel: w192 -> [w312]
      tunnel: w209 -> [w327]
      tunnel: w208 -> [w326]
      tunnel: w201 -> [w318]
      tunnel: w191 -> [w306]
      i -> [w374]
      stop <- w321 stop-if-true
      (unwired) u64 8323072 ("port")
      (unwired) i16 -16 ("y")
      n112 = Multiply(x=w374, y=16 ("length (rest)")) -> (x*y=w313:i32)
      n113 = local read "display"() -> (w350:bool)
      n114 = Add(x=w313, y=10 ("length (rest)")) -> (x+y=w340:i32)
      n115 = Add(x=w313, y=4 ("length (rest)")) -> (x+y=w315:i32)
      n116 = Add(x=w313, y=0 ("length (rest)")) -> (x+y=w324:i32)
      n117 = String Subset(string=w325, offset (0)=w324, length (rest)=16 ("y")) -> (substring=w322:string)
      n118 = String Subset(string=w325, offset (0)=w324, length (rest)=8 ("length (rest)")) -> (substring=w304:string)
      "substring" <- w304
      n119 = String Subset(string=w312, offset (0)=w340, length (rest)=6 ("length (rest)")) -> (substring=w300:string)
      "substring 2" <- w300
      n120 = String Subset(string=w312, offset (0)=w315, length (rest)=4 ("length (rest)")) -> (substring=w299:string)
      "substring 3" <- w299
      n121 = case shown="False" w350 {
        tunnel: w371 -> [_ w400]
        frame False {
        }
        frame True {
          n122 = Index Array(array=w400, index (col)="channel for cal") -> (element=→"cal":u32[])  [unwired: 1 in]
        }
      }
      n123 = String Length(string=w322) -> (length=w368:i32)
      n124 = Less?(x=w368, y=16) -> (x < y?=w321:bool)
      n125 = String Subset(string=w304, length (rest)=1 ("length (rest)")) -> (substring=w345:string)  [unwired: 1 in]
      n126 = String Subset(string=w304, offset (0)=5, length (rest)=2 ("length (rest)")) -> (substring=w328:string)
      n127 = String Subset(string=w304, offset (0)=2, length (rest)=1 ("length (rest)")) -> (substring=w302:string)
      n128 = Equal?(x=w345, y="Z" ("format string")) -> (x = y?=w330:bool)
      n129 = Equal?(x=w328, y=w306) -> (x = y?=w329:bool)
      n130 = String To Byte Array(string=w300) -> (unsigned byte array=w337:u8[])
      n131 = String To Byte Array(string=w299) -> (unsigned byte array=w308:u8[])
      n132 = String To Byte Array(string=w302) -> (unsigned byte array=w376:u8[])
      n133 = for {
        shift-right: [w588] -> w334
        shift-left: "" ("format string") -> [w585]
        tunnel: w376 -> [w589] mode=indexing
        n134 = Number To Hexadecimal String(2:w589) -> (0:w581:string)  [unwired: 1 in]
        n135 = String Length(string=w581) -> (length=w587:i32)
        n136 = Equal?(x=w587, y=2) -> (x = y?=w584:bool)
        n137 = Concatenate Strings("0" ("format string"), w581) -> (w583:string)
        n138 = Select(t=w581, s=w584, f=w583) -> (s? t:f=w580:string)
        n139 = Concatenate Strings(w585, w580) -> (w588:string)
      }
      n140 = for {
        shift-right: [w396] -> w335
        shift-left: "" ("format string") -> [w388]
        tunnel: w337 -> [w397] mode=indexing
        n141 = Number To Hexadecimal String(2:w397) -> (0:w390:string)  [unwired: 1 in]
        n142 = String Length(string=w390) -> (length=w395:i32)
        n143 = Concatenate Strings("0" ("format string"), w390) -> (w392:string)
        n144 = Equal?(x=w395, y=2) -> (x = y?=w393:bool)
        n145 = Select(t=w390, s=w393, f=w392) -> (s? t:f=w389:string)
        n146 = Concatenate Strings(w388, w389) -> (w396:string)
      }
      n147 = for {
        shift-right: [w386] -> w311
        shift-left: "" ("format string") -> [w378]
        tunnel: w308 -> [w387] mode=indexing
        n148 = Number To Hexadecimal String(2:w387) -> (0:w380:string)  [unwired: 1 in]
        n149 = String Length(string=w380) -> (length=w385:i32)
        n150 = Concatenate Strings("0" ("format string"), w380) -> (w382:string)
        n151 = Equal?(x=w385, y=2) -> (x = y?=w383:bool)
        n152 = Select(t=w380, s=w383, f=w382) -> (s? t:f=w379:string)
        n153 = Concatenate Strings(w378, w379) -> (w386:string)
      }
      n154 = Not(x=w321) -> (.not. x?=w320:bool)
      n155 = Compound Arithmetic op=AND(w330, w329, w320) -> (w343:bool)
      n156 = Hexadecimal String To Number(string=w334, default (0uL)=u64 0 ("default (0 U32)")) -> (number=w372:u64)  [unwired: 1 in, 1 out]
      n157 = Hexadecimal String To Number(string=w335, default (0uL)=u64 0 ("default (0 U32)")) -> (number=w333:u64)  [unwired: 1 in, 1 out]
      n158 = Hexadecimal String To Number(string=w311, default (0uL)=u64 0 ("default (0 U32)")) -> (number=w307:u64)  [unwired: 1 in, 1 out]
      n159 = And(x=w372, y=u64 127 ("port")) -> (x .and. y?=w301:u64)
      "channel number" <- w301
      n160 = Equal To 0?(x=w301) -> (x = 0?=w358:bool)
      n161 = Equal?(x=w301, y=u64 1) -> (x = y?=w356:bool)
      n162 = case shown="True" w343 {
        tunnel: w333 -> [_ w440]
        tunnel: w363 -> [w406 w430]
        tunnel: w371 -> [w409 w439]
        tunnel: [w409 w438] -> w373
        tunnel: [w408 w435] -> w369
        tunnel: w370 -> [w408 w434]
        tunnel: w301 -> [_ w414]
        tunnel: w365 -> [w407 w433]
        tunnel: [w407 w432] -> w366
        tunnel: [w406 w431] -> w364
        tunnel: w362 -> [w405 w429]
        tunnel: [w405 w428] -> w361
        tunnel: w358 -> [_ w427]
        tunnel: w355 -> [w404 w426]
        tunnel: [w404 w425] -> w357
        tunnel: w356 -> [_ w424]
        tunnel: w354 -> [w403 w423]
        tunnel: [w403 w422] -> w353
        tunnel: w319 -> [w402 w420]
        tunnel: [w402 w419] -> w351
        tunnel: w352 -> [_ w418]
        tunnel: w349 -> [w401 w416]
        tunnel: [w401 w415] -> w348
        tunnel: w327 -> [_ w413]
        tunnel: w326 -> [_ w412]
        tunnel: w318 -> [_ w411]
        tunnel: w307 -> [_ w410]
        frame False {
          (unwired) FALSE
        }
        frame True {
          (unwired) 100001 ("y")
          n163 = Index Array(array=w429, index=w414) -> (element=w421:u32)
          n164 = Greater?(x=w421, y=w411) -> (0:w417:bool)
          n165 = And(x=w440, y=u64 1023 ("port")) -> (x .and. y?=w436:u64)
          n166 = case shown="True" w417 {
            tunnel: w440 -> [_ w552]
            tunnel: w439 -> [w458 w538]
            tunnel: [w457 w538] -> w438
            tunnel: w436 -> [w449 w489]
            tunnel: [w456 w522] -> w435
            tunnel: w434 -> [w456 w545]
            tunnel: w430 -> [w454 _]
            tunnel: w414 -> [w452 w520]
            tunnel: w433 -> [w455 w544]
            tunnel: [w455 w543] -> w432
            tunnel: [w454 w541] -> w431
            tunnel: w421 -> [w450 _]
            tunnel: w429 -> [w453 w540]
            tunnel: [w451 w540] -> w428
            tunnel: w427 -> [_ w533]
            tunnel: w426 -> [w448 w532]
            tunnel: [w448 w531] -> w425
            tunnel: w424 -> [_ w530]
            tunnel: w423 -> [w447 w529]
            tunnel: [w447 w528] -> w422
            tunnel: w421 -> [w445 _]
            tunnel: w411 -> [w442 _]
            tunnel: w420 -> [w444 w524]
            tunnel: [w443 w524] -> w419
            tunnel: w418 -> [_ w523]
            tunnel: w416 -> [w441 w517]
            tunnel: [w441 w516] -> w415
            tunnel: w414 -> [_ w513]
            tunnel: w413 -> [_ w511]
            tunnel: w412 -> [_ w512]
            tunnel: w410 -> [_ w506]
            tunnel: w410 -> [_ w495]
            frame False {
              n167 = Equal?(x=w445, y=w442) -> (x = y?=w446:bool)
              n168 = case shown="True" w446 {
                tunnel: w458 -> [w469 w475]
                tunnel: [w467 w475] -> w457
                tunnel: w453 -> [w465 w473]
                tunnel: w452 -> [w464 w470]
                tunnel: [w462 w472] -> w451
                tunnel: w450 -> [w461 w471]
                tunnel: w449 -> [w460 _]
                tunnel: w444 -> [w459 w477]
                tunnel: [w459 w476] -> w443
                frame False {
                  n169 = Index Array(array=w469, index (row)=w460, index (col)=w464) -> (element=w468:u32)
                  n170 = Increment(x=w468) -> (x+1=w466:u32)
                  n171 = Replace Array Subset(array=w469, new element=w466, index (row)=w460, index (col)=w464) -> (w467:u32[][])
                  n172 = Increment(x=w461) -> (x+1=w463:u32)
                  n173 = Replace Array Subset(array=w465, new element=w463, index=w464) -> (w462:u32[])
                  "Calibration Counter" <- w461
                }
                frame True {
                  n174 = for {
                    N: 2048 -> [_]
                    tunnel: w475 -> [w487]
                    tunnel: w470 -> [w480]
                    shift-right: [w482] -> w476
                    shift-left: w477 -> [w483]
                    i -> [w479]
                    n175 = Array Subset(array=w487, index (row)=0 ("索引"), length (row)=w479, index (col)=w480, length (col)=1 ("长度")) -> (w484:u32[][])
                    n176 = Add Array Elements(numeric array=w484) -> (sum=w481:u32)
                    n177 = Replace Array Subset(array=w483, new element=w481, index (row)=w479, index (col)=w480) -> (w482:u32[][])
                  }
                  n178 = Increment(x=w471) -> (x+1=w474:u32)
                  n179 = Replace Array Subset(array=w473, new element=w474, index=w470) -> (w472:u32[])
                }
              }
            }
            frame True {
              (unwired) 0.0 ("x")
              w535 = 0 ("索引 (行)")
              w537 = 1 ("长度")
              # "正式取数"
              n180 = And(x=w495, y=u64 16711680 ("port")) -> (x .and. y?=w503:u64)
              n181 = And(x=w506, y=u64 4294967295 ("port")) -> (x .and. y?=w509:u64)
              n182 = Logical Shift(y=i16 -3, x=w509) -> (x << y=w490:u64)
              n183 = Logical Shift(y=i16 -32, x=w503) -> (x << y=w502:u64)
              n184 = And(x=w495, y=u64 255 ("port")) -> (x .and. y?=w494:u64)
              n185 = And(x=w552, y=u64 1099511626752 ("port")) -> (x .and. y?=w549:u64)
              n186 = Multiply(x=u64 3600, y=w502) -> (x*y=w498:u64)
              n187 = Multiply(x=u64 60, y=w490) -> (x*y=w499:u64)
              n188 = Logical Shift(y=i16 -11, x=w549) -> (x << y=w488:u64)
              "fine 2" <- w488
              n189 = Add(x=w499, y=w498) -> (x+y=w497:u64)
              n190 = Add(x=w497, y=w494) -> ()  [unwired: 1 out]
              n191 = Equal?(x=w513, y=u32 2) -> (x = y?=w515:bool)
              n192 = case shown="True" w515 {
                tunnel: w517 -> [w553 w556]
                tunnel: w488 -> [_ w555]
                tunnel: [w553 w554] -> w516
                frame False {
                }
                frame True {
                  n193 = Build Array (concatenate)(w556, w555) -> (w554:u64[])
                }
              }
              "cal 2" <- w516
              n194 = case shown="True" TRUE {
                tunnel: [w563 w571] -> w547
                tunnel: w538 -> [_ _]
                tunnel: w520 -> [w568 w569]
                tunnel: w489 -> [w566 w574]
                tunnel: w524 -> [w567 w575]
                frame False {
                  w562 = 0 ("index (row)")
                  w565 = 1 ("长度")
                  n195 = Decrement(x=w568) -> (x-1=w561:u64)
                  n196 = Array Subset(array=w567, index (row)=w566, length (row)=w565, index (col)=w561, length (col)=w565) -> (w564:u32[][])
                  n197 = Index Array(array=w564, index (row)=w562, index (col)=w562) -> (element=w563:u32)
                }
                frame True {
                  w570 = 0 ("index (row)")
                  w573 = 1 ("长度")
                  n198 = Array Subset(array=w575, index (row)=w574, length (row)=w573, index (col)=w569, length (col)=w573) -> (w572:u32[][])
                  n199 = Index Array(array=w572, index (row)=w570, index (col)=w570) -> (element=w571:u32)
                }
              }
              n200 = Multiply(x=w488, y=w511) -> (x*y=w493:dbl)
              n201 = Index Array(array=w544, index=w520) -> (element=w541:u32)
              n202 = Array Subset(array=w538, index (row)=w489, length (row)=w537, index (col)=w520, length (col)=w537) -> (w536:u32[][])
              n203 = Index Array(array=w536, index (row)=w535, index (col)=w535) -> (element=w534:u32)
              n204 = Divide(x=w534, y=u32 2) -> (x/y=w539:dbl)
              n205 = Increment(x=w541) -> (x+1=w542:u32)
              n206 = Add(x=w547, y=w539) -> (x+y=w546:dbl)
              n207 = Add(x=w493, y=0.0) -> (x+y=w492:dbl)
              n208 = Multiply(x=w546, y=w512) -> (x*y=w526:dbl)
              n209 = Subtract(x=w511, y=w526) -> (x-y=w510:dbl)
              n210 = Add(x=w510, y=w492) -> (x+y=w527:dbl)
              n211 = Replace Array Subset(array=w544, new element=w542, index=w520) -> (w543:u32[])
              n212 = case shown="True" w533 {
                tunnel: w527 -> [_ w579]
                tunnel: [w578 w579] -> w531
                tunnel: w532 -> [w578 _]
                frame False {
                }
                frame True {
                }
              }
              n213 = case shown="False" w530 {
                tunnel: [w576 w577] -> w528
                tunnel: w529 -> [w576 _]
                tunnel: w527 -> [_ w577]
                frame False {
                }
                frame True {
                }
              }
              n214 = Replace Array Subset(array=w545, new element=w527, index=w520) -> (w521:dbl[])
              n215 = case shown="True" "save data" {
                tunnel: w523 -> [_ w560]
                tunnel: w521 -> [_ w558]
                frame False {
                }
                frame True {
                  n216 = call-poly <vilib>:"Write Delimited Spreadsheet.vi"("file path (dialog if empty)"=w560, "1D data"=w558, "append to file? (new file:F)"="append csv", "delimiter (\\t)"="," ("delimiter (\\t)")) -> ()  [unwired: 10 in, 2 out]
                }
              }
              n217 = Replace Array Subset(array=w521, new element=0.0 ("new element/subarray"), index=w520) -> (w522:dbl[])
              "fine" <- w489
            }
          }
        }
      }
    }
    n218 = case shown="True" "RST" {
      tunnel: w199 -> [w296 _]
      tunnel: [w296 0] -> w227
      tunnel: [w295 w297] -> w225
      tunnel: w200 -> [w295 _]
      frame False {
      }
      frame True {
        n219 = Get Date/Time In Seconds() -> (seconds since 1Jan1904=w297:timestamp)
      }
    }
  }
  "error out 2" <- w47
  n220 = Close File(refnum=w24, error in=w88) -> (error out=→"error out":errorcluster)  [unwired: 1 out]
  n221 = call-poly <vilib>:"Write Delimited Spreadsheet.vi"("file path (dialog if empty)"=w60, "2D data"=w61, "append to file? (new file:F)"=FALSE, "transpose? (no:F)"=TRUE, "delimiter (\\t)"="," ("delimiter (\\t)")) -> ()  [unwired: 9 in, 2 out]
